vi "AcquireImage.vi"(2 "RO Done":bool, 4 "Acq Mode":T1 caption="Acquisition Mode", 5 "Save As":u16(ring) items=["U16 FITS", "I16 FITS", "I32 FITS", "SGL FITS", "U16 TIFF", "I16 TIFF", "I32 TIFF", "SGL TIFF"], 6 "Error in":errorcluster, 7 "File Name":string, 8 "Mode":u16(ring)=1 items=["Retrieve Image Buffer", "Acquire and transfer to client", "Acquire and hold in Server Image Buffer", "Acquire, transfer to client and save to Server's disk", "Acquire, save to Server's disk and hold in Server Image Buffer"], 9 "TCP/IP ID":refnum<k5>) -> (0 "Error out":errorcluster, 1 "% Complete":u16(slide) caption="% Readout" scale=0.0..100.0, 3 "% Exposure":u16(slide) scale=0.0..100.0)   [LabVIEW 2015]
uses:
  Client Acquisition Mode Menu.ctl
panel:
  in  "# to Average":u32=2 caption="of"
  out "Packet\nError code":i32
  out "Function #":u16
  out "Acquiring":u32
  out "Image":sgl[][](graph)
  out "S Len":i32
  out "P Len":i32
  in  "Acquire":bool
  out "Read String":string
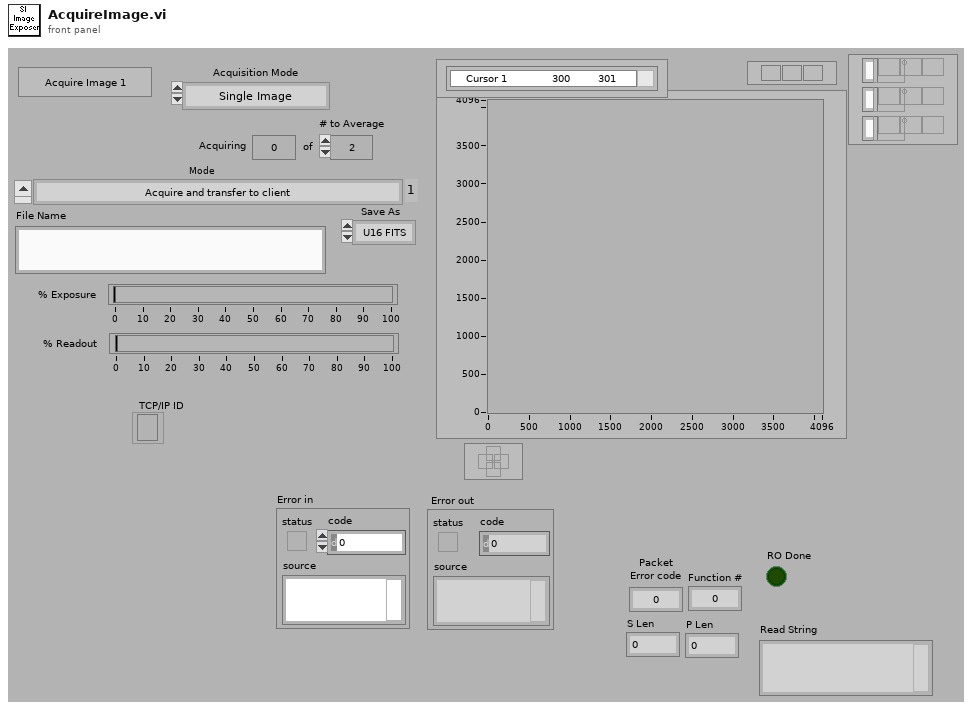
[diagram p1: front panel]
types:
  T1 = typedef "Client Acquisition Mode Menu.ctl" = enum16{"Single Image", "Average Images", "Multiple Frames"}
  T2 = cluster{"% Exp.":u16, "%Readout":u16, "Relative Pos.":u32, "Acquiring":dbl}
  T3 = typedef "TCP-IP Image Packet.ctl" = cluster{"Image ID":u16, "Image Type":u16, "Serial Length":u16, "Parallel Length":u16, "# of Packets":u16, "Packet #":u16, "Offset":u32, "Image Bytes":u32, "Image Data $":string}
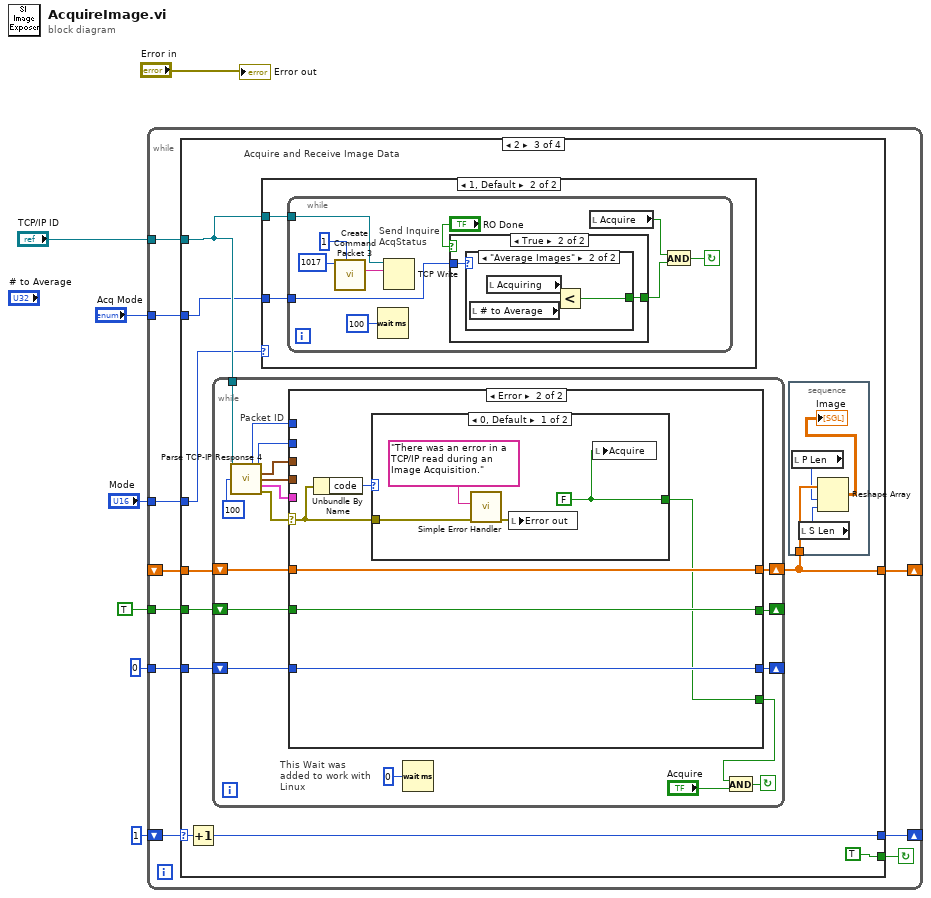
[diagram p0: block diagram]
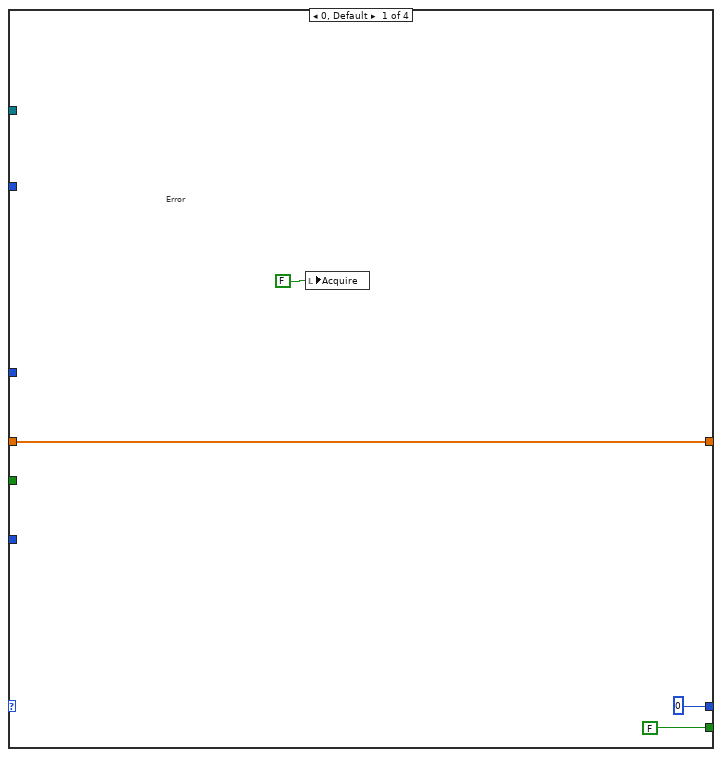
[diagram p2: hidden frame]
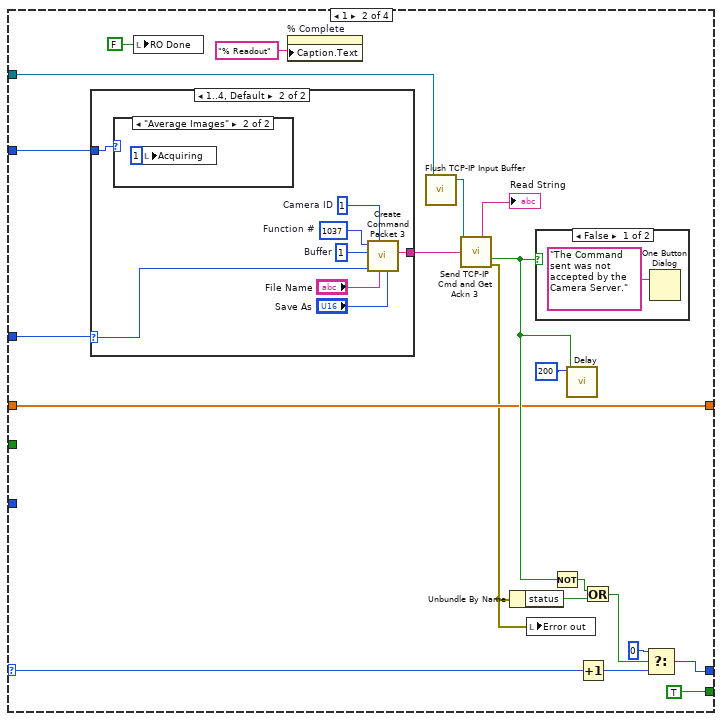
[diagram p3: hidden frame]
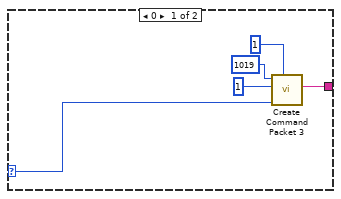
[diagram p4: hidden frame]
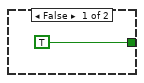
[diagram p8: hidden frame]
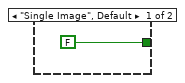
[diagram p9: hidden frame]
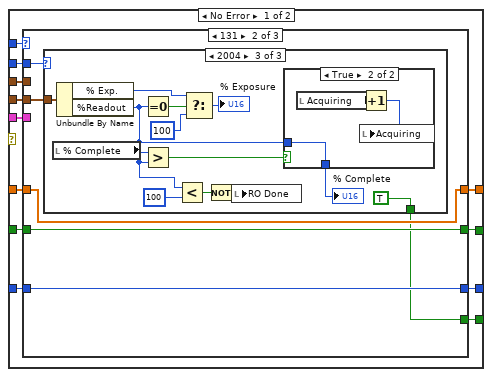
[diagram p10: hidden frame]
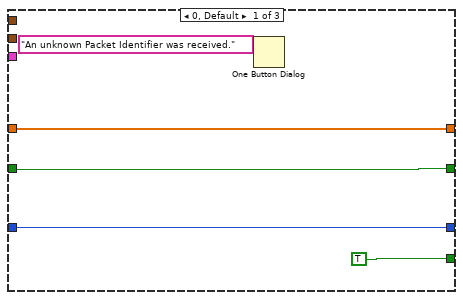
[diagram p11: hidden frame]
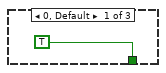
[diagram p12: hidden frame]
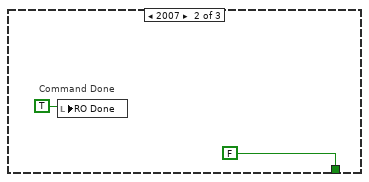
[diagram p13: hidden frame]
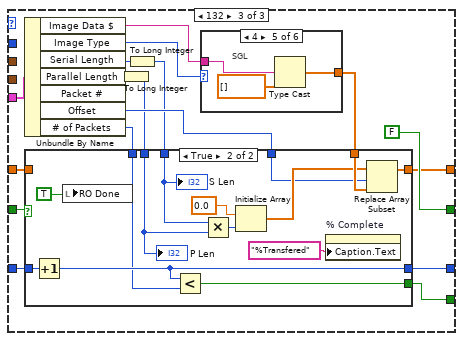
[diagram p15: hidden frame]
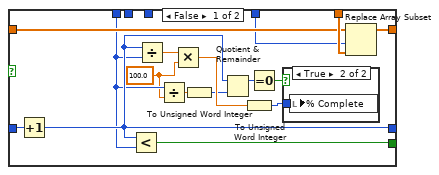
[diagram p16: hidden frame]
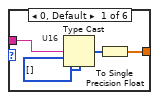
[diagram p18: hidden frame]
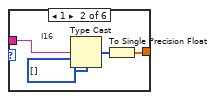
[diagram p19: hidden frame]
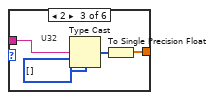
[diagram p20: hidden frame]
diagram:
  n1 = while {
    tunnel: u16 0 -> [w9]
    tunnel: TRUE -> [w10]
    shift-left: _ -> [w12]
    shift-right: [w11] -> _
    tunnel: "TCP/IP ID" -> [w13]
    tunnel: "Mode" -> [w14]
    shift-left: 1 -> [w17]
    shift-right: [w16] -> _
    tunnel: "Acq Mode" -> [w8]
    stop <- w15 continue-if-true
    n2 = case shown="2" w17 {
      selector: w17 -> [_ w41 w65 w240]
      tunnel: [0 w33 w66 w240] -> w16
      tunnel: [FALSE TRUE TRUE w235] -> w15
      tunnel: w14 -> [_ w27 w57 w238]
      tunnel: w13 -> [_ w39 w63 w239]
      tunnel: w12 -> [w18 w24 w62 w234]
      tunnel: [w18 w24 w59 w234] -> w11
      tunnel: w10 -> [_ _ w61 _]
      tunnel: w9 -> [_ _ w60 _]
      tunnel: w8 -> [_ w23 w58 w233]
      frame 0, Default {
        # "Error"
        n3 = local write "Acquire"(FALSE) -> ()
      }
      frame 1 {
        n4 = case shown="1..4, Default" w27 {
          selector: w27 -> [w43 w50]
          tunnel: [w44 w52] -> w37
          tunnel: w23 -> [_ w47]
          frame 0 {
            n5 = call "Create Command Packet 3.vi"("Camera ID (1)"=u8 1 ("Camera ID"), "Mode"=w43, "Buffer/Avg #/Frames"=u16 1 ("Buffer #"), "Function #"=u16 1019) -> ("Cmd Packet"=w44:string)  [unwired: 7 in]
          }
          frame 1..4, Default {
            w54 = u16 1037  # Function #
            w51 = u32 1  # Buffer
            w53 = u8 1  # Camera ID
            n6 = case shown="\"Average Images\"" w47 {
              frame "Single Image", Default {
              }
              frame "Average Images" {
                n7 = local write "Acquiring"(u32 1 ("Acquiring")) -> ()
              }
            }
            n8 = call "Create Command Packet 3.vi"("Save As"="Save As", "File Name"="File Name", "Camera ID (1)"=w53, "Mode"=w50, "Buffer/Avg #/Frames"=w51, "Function #"=w54) -> ("Cmd Packet"=w52:string)  [unwired: 5 in]
          }
        }
        n9 = local write "RO Done"(FALSE ("RO Done")) -> ()
        n10 = property on="% Complete" class="Slide (strict)"("Caption.Text"="% Readout") -> ()  [unwired: 2 in, 2 out]
        n11 = call "Flush TCP-IP Input Buffer.vi"("TCP/IP ID"=w39) -> ("TCP/IP ID Out"=w38:refnum<k5>)  [unwired: 4 in]
        n12 = call "Send TCP-IP Cmd and Get Ackn 3.vi"("TCP/IP ID In"=w38, "Cmd Packet"=w37) -> ("Read String"=→"Read String":string, "Accepted Flag"=w29:bool, "error out"=w22:errorcluster)  [unwired: 7 in, 4 out]
        n13 = Unbundle By Name(w22) -> ("status"=w36:bool)
        n14 = local write "Error out"(w22) -> ()
        n15 = case shown="False" w29 {
          frame False {
            n16 = One Button Dialog(message="The Command sent was not accepted by the Camera Server.") -> ()  [unwired: 1 in, 1 out]
          }
          frame True {
          }
        }
        n17 = Not(x=w29) -> (.not. x?=w31:bool)
        n18 = call "Delay.vi"("Boolean In"=w29, "milliseconds to wait (10)"=u32 200) -> ()  [unwired: 8 in, 2 out]
        n19 = Increment(x=w41) -> (x+1=w35:i32)
        n20 = Or(x=w31, y=w36) -> (x .or. y?=w32:bool)
        n21 = Select(t=0, s=w32, f=w35) -> (s? t:f=w33:i32)
      }
      frame 2 {
        # "Acquire and Receive Image Data"
        n22 = Increment(x=w65) -> (x+1=w66:i32)
        n23 = while {
          shift-left: w60 -> [w91]
          shift-right: [w90] -> _
          shift-left: w61 -> [w93]
          shift-right: [w92] -> _
          shift-left: w62 -> [w94]
          shift-right: [w88] -> w59
          tunnel: w63 -> [w103]
          stop <- w99 continue-if-true
          # "This Wait was added to work with Linux"
          # "Packet ID"
          n24 = call "Parse TCP-IP Response 4.vi"("TCP/IP ID"=w103, "timeout ms (5000)"=100) -> ("Packet ID"=w102:u8, "Data Type"=w96:u16, "Command Done"=w101:cluster{"Function #":u16}, "Acq. Status"=w100:T2, "Image Packet"=w95:T3, "error out"=w97:errorcluster)  [unwired: 3 in, 5 out]
          n25 = case shown="Error" w97 {
            selector: w97 -> [_ w218]
            tunnel: w102 -> [w115 _]
            tunnel: w101 -> [w114 _]
            tunnel: w100 -> [w113 _]
            tunnel: [w112 w219] -> w98
            tunnel: w96 -> [w111 _]
            tunnel: w95 -> [w110 _]
            tunnel: w94 -> [w109 w222]
            tunnel: [w108 w222] -> w88
            tunnel: w93 -> [w107 w223]
            tunnel: [w106 w223] -> w92
            tunnel: w91 -> [w105 w221]
            tunnel: [w104 w221] -> w90
            frame No Error {
              n26 = case shown="131" w115 {
                tunnel: w114 -> [_ _ _]
                tunnel: w113 -> [_ w126 _]
                tunnel: [TRUE w121 w151] -> w112
                tunnel: w111 -> [_ w123 _]
                tunnel: w110 -> [_ _ w159]
                tunnel: w109 -> [w116 w122 w150]
                tunnel: [w116 w122 w154] -> w108
                tunnel: w107 -> [w119 w125 w149]
                tunnel: [w119 w125 FALSE] -> w106
                tunnel: w105 -> [w118 w124 w153]
                tunnel: [w118 w124 w152] -> w104
                frame 0, Default {
                  n27 = One Button Dialog(message="An unknown Packet Identifier was received.") -> ()  [unwired: 1 in, 1 out]
                }
                frame 131 {
                  n28 = case shown="2004" w123 {
                    tunnel: w126 -> [_ _ w142]
                    tunnel: [TRUE FALSE TRUE] -> w121
                    frame 0, Default {
                    }
                    frame 2007 {
                      # "Command Done"
                      n29 = local write "RO Done"(TRUE) -> ()
                    }
                    frame 2004 {
                      n30 = local read "% Complete"() -> (w136:u16)
                      n31 = Unbundle By Name(w142) -> ("% Exp."=w131:u16, "%Readout"=w134:u16)
                      n32 = Equal To 0?(x=w134) -> (x = 0?=w133:bool)
                      n33 = Greater?(x=w136, y=w134) -> (0:w135:bool)
                      n34 = Less?(x=w134, y=u16 100) -> (x < y?=w140:bool)
                      n35 = Select(t=w131, s=w133, f=u16 100) -> (s? t:f=→"% Exposure":u16)
                      n36 = Not(x=w140) -> (.not. x?=w139:bool)
                      n37 = local write "RO Done"(w139) -> ()
                      n38 = case shown="True" w135 {
                        tunnel: [w143 w144] -> w137
                        tunnel: w134 -> [w143 w144]
                        frame False {
                        }
                        frame True {
                          n39 = local read "Acquiring"() -> (w145:u32)
                          n40 = Increment(x=w145) -> (x+1=w146:u32)
                          n41 = local write "Acquiring"(w146) -> ()
                        }
                      }
                      "% Complete" <- w137
                    }
                  }
                }
                frame 132 {
                  n42 = Unbundle By Name(w159) -> ("Image Data $"=w162:string, "Image Type"=w161:u16, "Serial Length"=w158:u16, "Parallel Length"=w157:u16, "Offset"=w156:u32, "# of Packets"=w160:u16)  [unwired: 1 out]
                  n43 = To Long Integer(number=w157) -> (32bit integer=w147:i32)
                  n44 = To Long Integer(number=w158) -> (32bit integer=w148:i32)
                  n45 = case shown="4" w161 {
                    tunnel: [w197 w200 w205 w208 w212 w215] -> w155
                    tunnel: w162 -> [w195 w199 w203 w207 w211 w214]
                    frame 0, Default {
                      # "U16"
                      n46 = Type Cast(type=u16[] [] ("Array Constant"), x=w195) -> (*(type *) &x=w198:u16[])
                      n47 = To Single Precision Float(number=w198) -> (single precision float=w197:sgl[])
                    }
                    frame 1 {
                      # "I16"
                      n48 = Type Cast(type=i16[] [] ("Array Constant"), x=w199) -> (*(type *) &x=w202:i16[])
                      n49 = To Single Precision Float(number=w202) -> (single precision float=w200:sgl[])
                    }
                    frame 2 {
                      # "U32"
                      n50 = Type Cast(type=u32[] [] ("Array Constant"), x=w203) -> (*(type *) &x=w206:u32[])
                      n51 = To Single Precision Float(number=w206) -> (single precision float=w205:sgl[])
                    }
                    frame 3 {
                      # "I32"
                      n52 = Type Cast(type=i32[] [] ("Array Constant"), x=w207) -> (*(type *) &x=w210:i32[])
                      n53 = To Single Precision Float(number=w210) -> (single precision float=w208:sgl[])
                    }
                    frame 4 {
                      # "SGL"
                      n54 = Type Cast(type=sgl[] [] ("Array Constant"), x=w211) -> (*(type *) &x=w212:sgl[])
                    }
                    frame 5 {
                      # "DBL"
                      n55 = Type Cast(type=dbl[] [] ("Array Constant"), x=w214) -> (*(type *) &x=w217:dbl[])
                      n56 = To Single Precision Float(number=w217) -> (single precision float=w215:sgl[])
                    }
                  }
                  n57 = case shown="True" w149 {
                    tunnel: w150 -> [w170 _]
                    tunnel: w148 -> [_ w182]
                    tunnel: w147 -> [_ w181]
                    tunnel: [w171 w193] -> w154
                    tunnel: w155 -> [w179 w192]
                    tunnel: w153 -> [w178 w190]
                    tunnel: [w168 w189] -> w152
                    tunnel: [w177 w188] -> w151
                    tunnel: w156 -> [w169 w185]
                    tunnel: w160 -> [w166 w184]
                    frame False {
                      w165 = 100.0 ("y")
                      n58 = Increment(x=w178) -> (x+1=w168:u16)
                      n59 = Less?(x=w168, y=w166) -> (x < y?=w177:bool)
                      n60 = Divide(x=w168, y=w166) -> (x/y=w173:dbl)
                      n61 = Divide(x=w166, y=w165) -> (x/y=w167:dbl)
                      n62 = Multiply(x=w173, y=w165) -> (x*y=w172:dbl)
                      n63 = To Unsigned Word Integer(number=w167) -> (unsigned 16bit integer=w164:u16)
                      n64 = Quotient & Remainder(x=w168, y=w164) -> (x-y*floor(x/y)=w176:u16)  [unwired: 1 out]
                      n65 = To Unsigned Word Integer(number=w172) -> (unsigned 16bit integer=w174:u16)
                      n66 = Equal To 0?(x=w176) -> (x = 0?=w175:bool)
                      n67 = case shown="True" w175 {
                        tunnel: w174 -> [_ w180]
                        frame False {
                        }
                        frame True {
                          n68 = local write "% Complete"(w180) -> ()
                        }
                      }
                      n69 = Replace Array Subset(array=w170, new element=w179, index=w169) -> (w171:sgl[])
                    }
                    frame True {
                      n70 = Increment(x=w190) -> (x+1=w189:u16)
                      n71 = local write "RO Done"(TRUE) -> ()
                      n72 = Less?(x=w189, y=w184) -> (x < y?=w188:bool)
                      n73 = Multiply(x=w182, y=w181) -> (x*y=w186:i32)
                      n74 = Initialize Array(sgl 0.0 ("Element Data"), w186) -> (w191:sgl[])
                      n75 = property on="% Complete" class="Slide (strict)"("Caption.Text"="%Transfered") -> ()  [unwired: 2 in, 2 out]
                      n76 = Replace Array Subset(array=w191, new element=w192, index=w185) -> (w193:sgl[])
                      "S Len" <- w182
                      "P Len" <- w181
                    }
                  }
                }
              }
            }
            frame Error {
              n77 = Unbundle By Name(w218) -> ("code"=w220:i32)
              n78 = case shown="0, Default" w220 {
                tunnel: w218 -> [w227 _]
                tunnel: [w225 TRUE] -> w219
                frame 0, Default {
                  w225 = FALSE
                  n79 = call <vilib>:"Simple Error Handler.vi"("error source (\" \")"="There was an error in a TCP/IP read during an Image Acquisition.", "error in (no error)"=w227) -> ("error out"=w224:errorcluster)  [unwired: 3 in, 4 out]
                  n80 = local write "Error out"(w224) -> ()
                  n81 = local write "Acquire"(w225) -> ()
                }
                frame 56 {
                  # "Timeout -  Keep going"
                }
              }
            }
          }
          n82 = Wait (ms)(milliseconds to wait=u32 0) -> ()  [unwired: 1 out]
          n83 = And(x=w98, y="Acquire") -> (x .and. y?=w99:bool)
        }
        n84 = case shown="1, Default" w57 {
          tunnel: w63 -> [_ w68]
          tunnel: w58 -> [_ w67]
          frame 0 {
          }
          frame 1, Default {
            n85 = while {
              tunnel: w68 -> [w75]
              tunnel: w67 -> [w69]
              stop <- w73 continue-if-true
              # "Send Inquire\nAcqStatus"
              n86 = call "Create Command Packet 3.vi"("Camera ID (1)"=u8 1 ("Camera ID"), "Function #"=u16 1017) -> ("Cmd Packet"=w76:string)  [unwired: 9 in]
              n87 = Wait (ms)(milliseconds to wait=u32 100) -> ()  [unwired: 1 out]
              n88 = TCP Write(connection ID=w75, data in=w76) -> ()  [unwired: 2 in, 3 out]
              n89 = case shown="True" "RO Done" {
                tunnel: [TRUE w81] -> w72
                tunnel: w69 -> [_ w80]
                frame False {
                }
                frame True {
                  n90 = case shown="\"Average Images\"" w80 {
                    tunnel: [FALSE w83] -> w81
                    frame "Single Image", Default {
                    }
                    frame "Average Images" {
                      n91 = local read "# to Average"() -> (w84:u32)
                      n92 = local read "Acquiring"() -> (w85:u32)
                      n93 = Less?(x=w85, y=w84) -> (x < y?=w83:bool)
                    }
                  }
                }
              }
              n94 = local read "Acquire"() -> (w70:bool)
              n95 = And(x=w70, y=w72) -> (x .and. y?=w73:bool)
            }
          }
        }
        n96 = stacked-sequence {
          tunnel: w59 -> [w232]
          frame #0 {
            n97 = local read "P Len"() -> (w231:i32)
            n98 = local read "S Len"() -> (w230:i32)
            n99 = Reshape Array(w232, w231, w230) -> (→"Image":sgl[][])
          }
        }
      }
      frame 3 {
        w235 = FALSE
        n100 = case shown="1, Default" w238 {
          selector: w238 -> [w242 w251 w265]
          tunnel: w239 -> [_ w252 _]
          tunnel: [w242 w251 w265] -> w236
          tunnel: w233 -> [_ w245 _]
          frame 0 {
          }
          frame 1, Default {
            # "If Exposure was not 100%, acquisition was terminated so send TerminateAcquisition command."
            n101 = Equal?(x=w245, y=Client_Acquisition_Mode_Menu."Average Images") -> (x = y?=w243:bool)
            n102 = local read "# to Average"() -> (w249:u32)
            n103 = local read "% Exposure"() -> (w254:u16)
            n104 = local read "Acquiring"() -> (w250:u32)
            n105 = Less?(x=w250, y=w249) -> (x < y?=w248:bool)
            n106 = Less?(x=w254, y=u16 100) -> (x < y?=w247:bool)
            n107 = Select(t=w248, s=w243, f=w247) -> (s? t:f=w246:bool)
            n108 = case shown="True" w246 {
              tunnel: w252 -> [_ w263]
              frame False {
              }
              frame True {
                n109 = call "Create Command Packet 3.vi"("Camera ID (1)"=u8 1 ("Camera ID"), "Function #"=u16 1018) -> ("Cmd Packet"=w261:string)  [unwired: 9 in]
                n110 = call "Flush TCP-IP Input Buffer.vi"("TCP/IP ID"=w263) -> ("TCP/IP ID Out"=w257:refnum<k5>)  [unwired: 4 in]
                n111 = TCP Write(connection ID=w257, data in=w261) -> (error out=w260:errorcluster)  [unwired: 2 in, 2 out]
                n112 = call "Parse TCP-IP Response 4.vi"("TCP/IP ID"=w257, "error in (no error)"=w260) -> ("Packet Error Code"=→"Packet\nError code":i32, "Command Done"=w259:cluster{"Function #":u16}, "error out"=w255:errorcluster)  [unwired: 3 in, 8 out]
                n113 = Unbundle By Name(w259) -> ("Function #"=→"Function #":u16)
                n114 = local write "Error out"(w255) -> ()
              }
            }
          }
          frame 5 {
          }
        }
        n115 = stacked-sequence {
          tunnel: w236 -> [_]
          frame #0 {
            w241 = u16 0 ("% Exposure")
            n116 = local write "% Exposure"(w241) -> ()
            n117 = local write "% Complete"(w241) -> ()
            "Acquiring" <- w241
          }
        }
        n118 = property on="% Complete" class="Slide (strict)"("Caption.Text"="% Readout") -> ()  [unwired: 2 in, 2 out]
        n119 = local write "Acquire"(w235) -> ()
      }
    }
  }
  "Error out" <- "Error in"
